vi "BuildMenu5 1.vi"(0 "XRef":T7, 1 "MenuRef":T6, 2 "Point":T4, 3 "Menu Type":T3, 4 "State In":T2) -> (14 "Fatal Error Out":T1)   [LabVIEW 2013, in "VireoFunctionNode.xnode"]
uses:
  VireoFunctionNode.xnode
  <vilib>/XNodeSupport/XNodeXNodeRef.ctl
  <vilib>/XNodeSupport/NI_XNodeSupport.lvlib
  <vilib>/XNodeSupport/XNodeMenuRef.ctl
  <vilib>/XNodeSupport/XNodeInt.ctl
  <vilib>/XNodeSupport/XNodePoint.ctl
  <vilib>/XNodeSupport/XNodeMenuType.ctl
  <vilib>/XNodeSupport/XNodeErrorCluster.ctl
  State 1.ctl
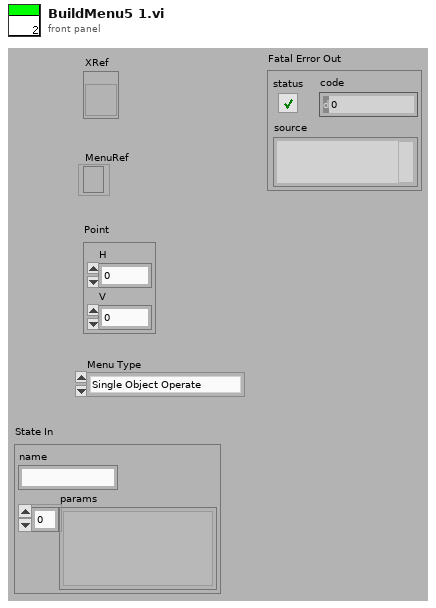
[diagram p1: front panel]
types:
  T1 = typedef "NI_XNodeSupport.lvlib/XNodeErrorCluster.ctl" = errorcluster
  T2 = typedef "VireoFunctionNode.xnode/State 1.ctl" = cluster{"name":string, "params":variant[]}
  T3 = typedef "NI_XNodeSupport.lvlib/XNodeMenuType.ctl" = enum32{"Single Object Operate", "Single Object Popup", "Multi Object Popup Master", "Multi Object Popup Other"}
  T4 = typedef "NI_XNodeSupport.lvlib/XNodePoint.ctl" = cluster{"H":T5, "V":T5}
  T5 = typedef "NI_XNodeSupport.lvlib/XNodeInt.ctl" = i32
  T6 = typedef "NI_XNodeSupport.lvlib/XNodeMenuRef.ctl" = refnum<k9>
  T7 = typedef "NI_XNodeSupport.lvlib/XNodeXNodeRef.ctl" = refnum<vi>
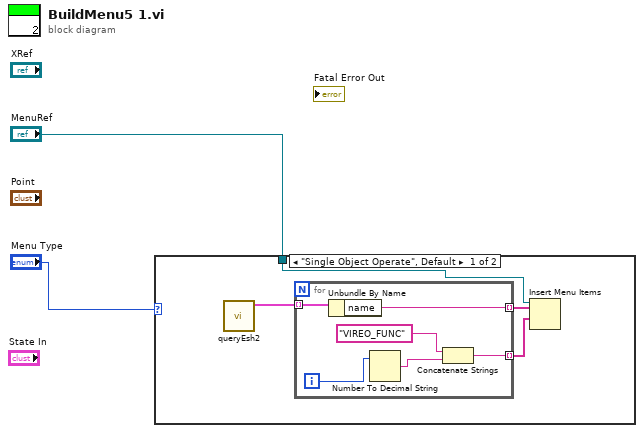
[diagram p0: block diagram]
diagram:
  n1 = case shown="\"Single Object Operate\", Default" "Menu Type" {
    tunnel: "MenuRef" -> [w4 _]
    frame "Single Object Operate", Default {
      n2 = call "queryEsh2.vi"() -> ("Array"=w6:cluster{"name":string, "params":variant[]}[])  [unwired: 11 in]
      n3 = for {
        tunnel: w6 -> [w12] mode=indexing
        tunnel: [w11] -> w5 mode=indexing
        tunnel: [w7] -> w3 mode=indexing
        i -> [w10]
        n4 = Unbundle By Name(w12) -> ("name"=w11:string)
        n5 = Number To Decimal String(number=w10) -> (decimal integer string=w9:string)  [unwired: 1 in]
        n6 = Concatenate Strings("VIREO_FUNC", w9) -> (w7:string)
      }
      n7 = Insert Menu Items(7:w3, 8:w5, 9:w4) -> ()  [unwired: 3 in, 3 out]
    }
    frame "Single Object Popup" {
    }
  }
